vi "CenToFa.vi"(11 "Grados C":dbl) -> (3 "Grados F":dbl)   [LabVIEW 2020]
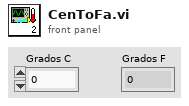
[diagram p1: front panel]
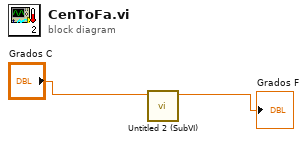
[diagram p0: block diagram]
diagram:
  n1 = call "Untitled 2 (SubVI).vi"("Grados C"="Grados C") -> ("Grados F"=→"Grados F":dbl)  [unwired: 10 in]
